vi "VisorTDMS.vi"() -> ()   [LabVIEW 2018]
uses:
  <vilib>/express/express shared/transition.llb/Dynamic To Waveform Array.vi
  <vilib>/express/express signal manip/GetorSetDDTAttributes/Set DDT Attributes/SetT0.vi
  <vilib>/express/express shared/transition.llb/Waveform Array To Dynamic.vi
  <vilib>/express/express signal manip/GetorSetDDTAttributes/Set DDT Attributes/Set DDT Properties.xnode
panel:
  out "fin_video":timestamp
  out "incio_video":timestamp
  out "is_altitude":string
  out "is_heading":string
  out "is_roll":string
  out "is_pitch":string
  out "is_depth":string
  out "is_gps_lon":string
  out "is_gps_lat":string
  out "Frame actual":i64
  in  "Frame-":bool
  in  "Frame+":bool
  in  "Retroceder":bool
  in  "Avanzar":bool
  in  "Mover Frame":i64
  in  "Tab Control":enum32{"TopData", "SubData"}(tab)
  in  "Tab Control 2":T1(tab)
  out "rov_states 2":dbl[](array[numeric])
  out "ind.":dbl[](array[numeric])
  out "modo_ctrl 2":dbl[](array[numeric])
  out "ac_time_TopData":timestamp[](array[timestamp])
  out "gps_alt":dbl[](array[numeric])
  out "usbl_x":dbl[](array[numeric])
  out "usbl_y":dbl[](array[numeric])
  out "usbl_z":dbl[](array[numeric])
  out "vess_ahrs_pitch":dbl[](array[numeric])
  out "vess_ahrs_roll":dbl[](array[numeric])
  out "vess_ahrs_yaw":dbl[](array[numeric])
  out "acquisition_time 5":timestamp[](array[timestamp])
  out "ci_habilitada":dbl[](array[numeric])
  out "CI_Data_joy_1x":dbl[](array[numeric])
  out "CI_Data_jot_1y":dbl[](array[numeric])
  out "CI_Data_jot_1z":dbl[](array[numeric])
  out "CI_Data_joy_1thumb":dbl[](array[numeric])
  out "CI_Data_joy_1botIzq":dbl[](array[numeric])
  out "CI_Data_joy_1botder":dbl[](array[numeric])
  out "acquisition_time 12":timestamp[](array[timestamp])
  out "CI_Data_joy_1gatillo":dbl[](array[numeric])
  out "CI_Data_modo_1bot":dbl[](array[numeric])
  out "CI_Data_modo_2bot":dbl[](array[numeric])
  out "CI_Data_modo_3bot":dbl[](array[numeric])
  out "CI_Data_modo_4bot":dbl[](array[numeric])
  out "CI_Data_pot":dbl[](array[numeric])
  out "CI_Data_enc":dbl[](array[numeric])
  out "CI_Data_joy_2x":dbl[](array[numeric])
  out "CI_Data_joy_2y":dbl[](array[numeric])
  out "CI_Data_joy_2z":dbl[](array[numeric])
  out "CI_Data_joy_2bot":dbl[](array[numeric])
  out "CI_Data_botella_1bot":dbl[](array[numeric])
  out "CI_Data_botella_2bot":dbl[](array[numeric])
  out "CI_Data_botella_3bot":dbl[](array[numeric])
  out "CI_Data_botella_4bot":dbl[](array[numeric])
  out "CI_Data_corer_1bot":dbl[](array[numeric])
  out "CI_Data_corer_2bot":dbl[](array[numeric])
  out "CI_Data_a_in":dbl[](array[numeric])
  out "CI_Data_dio1":dbl[](array[numeric])
  out "CI_Data_dio2":dbl[](array[numeric])
  out "CI_Data_dio3":dbl[](array[numeric])
  out "CI_Data_ci_acc_x":dbl[](array[numeric])
  out "CI_Data_ci_acc_y":dbl[](array[numeric])
  out "CI_Data_ci_acc_z":dbl[](array[numeric])
  out "Surface_Data_modo_1ind":dbl[](array[numeric])
  out "Surface_Data_modo_2ind":dbl[](array[numeric])
  out "Surface_Data_modo_3ind":dbl[](array[numeric])
  out "Surface_Data_modo_4ind":dbl[](array[numeric])
  out "Surface_Data_botella_1ind":dbl[](array[numeric])
  out "Surface_Data_botella_2ind":dbl[](array[numeric])
  out "Surface_Data_botella_3ind":dbl[](array[numeric])
  out "Surface_Data_botella_4ind":dbl[](array[numeric])
  out "Surface_Data_corer_1ind":dbl[](array[numeric])
  out "Surface_Data_corer_2ind":dbl[](array[numeric])
  out "Surface_Data_lars_vel":dbl[](array[numeric])
  out "Surface_Data_lars_fwd":dbl[](array[numeric])
  out "Surface_Data_lars_rev":dbl[](array[numeric])
  out "acquisition_time 13":timestamp[](array[timestamp])
  out "m1_hi":dbl[](array[numeric])
  out "m1_lo":dbl[](array[numeric])
  out "m1_en":dbl[](array[numeric])
  out "m2_hi":dbl[](array[numeric])
  out "m2_lo":dbl[](array[numeric])
  out "m2_en":dbl[](array[numeric])
  out "m3_hi":dbl[](array[numeric])
  out "m3_lo":dbl[](array[numeric])
  out "m3_en":dbl[](array[numeric])
  out "m4_hi":dbl[](array[numeric])
  out "m4_lo":dbl[](array[numeric])
  out "m4_en":dbl[](array[numeric])
  out "m5_hi":dbl[](array[numeric])
  out "m5_lo":dbl[](array[numeric])
  out "m5_en":dbl[](array[numeric])
  out "m6_hi":dbl[](array[numeric])
  out "m6_lo":dbl[](array[numeric])
  out "m6_en":dbl[](array[numeric])
  out "motor_PID_Kp":dbl[](array[numeric])
  out "motor_PID_Ti":dbl[](array[numeric])
  out "motor_PID_Td":dbl[](array[numeric])
  out "m_PID_en":dbl[](array[numeric])
  out "depth_PID_Kp":dbl[](array[numeric])
  out "depth_PID_Ti":dbl[](array[numeric])
  out "depth_PID_Td":dbl[](array[numeric])
  out "depth_sp":dbl[](array[numeric])
  out "heading_PID_Kp":dbl[](array[numeric])
  out "heading_PID_Ti":dbl[](array[numeric])
  out "heading_PID_Td":dbl[](array[numeric])
  out "heading_sp":dbl[](array[numeric])
  out "altitude_PID_Kp":dbl[](array[numeric])
  out "altitude_PID_Ti":dbl[](array[numeric])
  out "altitude_PID_Td":dbl[](array[numeric])
  out "altitude_sp":dbl[](array[numeric])
  out "PID_reset":dbl[](array[numeric])
  out "modo_ctrl":dbl[](array[numeric])
  out "bus_260v":dbl[](array[numeric])
  out "m_1":dbl[](array[numeric])
  out "m_2":dbl[](array[numeric])
  out "m_3":dbl[](array[numeric])
  out "m_4":dbl[](array[numeric])
  out "m_5":dbl[](array[numeric])
  out "m_6":dbl[](array[numeric])
  out "luz_1":dbl[](array[numeric])
  out "luz_2":dbl[](array[numeric])
  out "luz_3":dbl[](array[numeric])
  out "pot_gen":dbl[](array[numeric])
  out "pot_m1":dbl[](array[numeric])
  out "pot_m2":dbl[](array[numeric])
  out "pot_m3":dbl[](array[numeric])
  out "pot_m4":dbl[](array[numeric])
  out "pot_m5":dbl[](array[numeric])
  out "pot_m6":dbl[](array[numeric])
  out "pot_l1":dbl[](array[numeric])
  out "pot_l2":dbl[](array[numeric])
  out "pot_l3":dbl[](array[numeric])
  out "virtual_ci":dbl[](array[numeric])
  out "fuente_muestras":dbl[](array[numeric])
  out "corer_1":dbl[](array[numeric])
  out "corer_2":dbl[](array[numeric])
  out "bot_1":dbl[](array[numeric])
  out "bot_2":dbl[](array[numeric])
  out "bot_3":dbl[](array[numeric])
  out "bot_4":dbl[](array[numeric])
  out "pot_c1":dbl[](array[numeric])
  out "pot_c2":dbl[](array[numeric])
  out "acquisition_time 14":timestamp[](array[timestamp])
  in  "Tab Control 3":T2(tab)
  out "ac_time_SubData":timestamp[](array[timestamp])
  out "sub_ind":dbl[](array[numeric])
  out "sc_ind":dbl[](array[numeric])
  out "rov_states":dbl[](array[numeric])
  out "accel_x":dbl[](array[numeric])
  out "accel_y":dbl[](array[numeric])
  out "accel_z":dbl[](array[numeric])
  out "gyr_x":dbl[](array[numeric])
  out "acquisition_time 2":timestamp[](array[timestamp])
  out "gyr_y":dbl[](array[numeric])
  out "gyr_z":dbl[](array[numeric])
  out "mag_x":dbl[](array[numeric])
  out "mag_y":dbl[](array[numeric])
  out "mag_z":dbl[](array[numeric])
  out "acquisition_time 4":timestamp[](array[timestamp])
  out "pressure 4":dbl[](array[numeric])
  out "temperature 4":dbl[](array[numeric])
  out "conductivity":dbl[](array[numeric])
  out "density":dbl[](array[numeric])
  out "salinity":dbl[](array[numeric])
  out "speed_of_sound":dbl[](array[numeric])
  out "acquisition_time 3":timestamp[](array[timestamp])
  out "acquisition_time 6":timestamp[](array[timestamp])
  out "liquid_smp1":dbl[](array[numeric])
  out "liquid_smp2":dbl[](array[numeric])
  out "liquid_smp3":dbl[](array[numeric])
  out "liquid_smp4":dbl[](array[numeric])
  out "solid_smp1":dbl[](array[numeric])
  out "solid_smp2":dbl[](array[numeric])
  out "supply_12V":dbl[](array[numeric])
  out "motor_signal1":dbl[](array[numeric])
  out "motor_signal2":dbl[](array[numeric])
  out "cur_liq_1":dbl[](array[numeric])
  out "cur_liq_2":dbl[](array[numeric])
  out "ac_status":dbl[](array[numeric])
  out "voltaje_hvdc":dbl[](array[numeric])
  out "current_hvdc":dbl[](array[numeric])
  out "light1":dbl[](array[numeric])
  out "light2":dbl[](array[numeric])
  out "ligth_sphere":dbl[](array[numeric])
  out "voltage_l1_l2":dbl[](array[numeric])
  out "voltage_l2_l3":dbl[](array[numeric])
  out "voltage_l1_l3":dbl[](array[numeric])
  out "current_l1":dbl[](array[numeric])
  out "current_l2":dbl[](array[numeric])
  out "current_l3":dbl[](array[numeric])
  out "acquisition_time 7":timestamp[](array[timestamp])
  out "current_lights":dbl[](array[numeric])
  out "temp_ac_filter":dbl[](array[numeric])
  out "MA_1_status":dbl[](array[numeric])
  out "MA_1_ctr_signal":dbl[](array[numeric])
  out "MA_1_current":dbl[](array[numeric])
  out "MA_1_speed":dbl[](array[numeric])
  out "MA_2_status":dbl[](array[numeric])
  out "MA_2_ctr_signal":dbl[](array[numeric])
  out "MA_2_current":dbl[](array[numeric])
  out "MA_2_speed":dbl[](array[numeric])
  out "MA_3_status":dbl[](array[numeric])
  out "MA_3_ctr_signal":dbl[](array[numeric])
  out "MA_3_current":dbl[](array[numeric])
  out "MA_3_speed":dbl[](array[numeric])
  out "MA_4_status":dbl[](array[numeric])
  out "MA_4_ctr_signal":dbl[](array[numeric])
  out "MA_4_current":dbl[](array[numeric])
  out "MA_4_speed":dbl[](array[numeric])
  out "MA_5_status":dbl[](array[numeric])
  out "MA_5_ctr_signal":dbl[](array[numeric])
  out "MA_5_current":dbl[](array[numeric])
  out "MA_5_speed":dbl[](array[numeric])
  out "MA_6_status":dbl[](array[numeric])
  out "MA_6_ctr_signal":dbl[](array[numeric])
  out "MA_6_current":dbl[](array[numeric])
  out "MA_6_speed":dbl[](array[numeric])
  out "mode":dbl[](array[numeric])
  out "start":dbl[](array[numeric])
  out "lps":dbl[](array[numeric])
  out "controller":dbl[](array[numeric])
  out "voltage":dbl[](array[numeric])
  out "current":dbl[](array[numeric])
  out "temperature":dbl[](array[numeric])
  out "humidity":dbl[](array[numeric])
  out "leak":dbl[](array[numeric])
  out "pressure":dbl[](array[numeric])
  out "acquisition_time 8":timestamp[](array[timestamp])
  out "mode 2":dbl[](array[numeric])
  out "start 2":dbl[](array[numeric])
  out "lps 2":dbl[](array[numeric])
  out "controller 2":dbl[](array[numeric])
  out "voltage 2":dbl[](array[numeric])
  out "current 2":dbl[](array[numeric])
  out "temperature 2":dbl[](array[numeric])
  out "humidity 2":dbl[](array[numeric])
  out "leak 2":dbl[](array[numeric])
  out "pressure 2":dbl[](array[numeric])
  out "acquisition_time 9":timestamp[](array[timestamp])
  out "mode 3":dbl[](array[numeric])
  out "start 3":dbl[](array[numeric])
  out "lps 3":dbl[](array[numeric])
  out "controller 3":dbl[](array[numeric])
  out "voltage 3":dbl[](array[numeric])
  out "current 3":dbl[](array[numeric])
  out "temperature 3":dbl[](array[numeric])
  out "humidity 3":dbl[](array[numeric])
  out "leak 3":dbl[](array[numeric])
  out "pressure 3":dbl[](array[numeric])
  out "acquisition_time 10":timestamp[](array[timestamp])
  out "ctrl_state":dbl[](array[numeric])
  out "rov_output_x":dbl[](array[numeric])
  out "rov_output_y":dbl[](array[numeric])
  out "rov_output_z":dbl[](array[numeric])
  out "rov_output_yaw":dbl[](array[numeric])
  out "dac_outputs":dbl[](array[numeric])
  out "in_range":dbl[](array[numeric])
  out "motor_ctrl_array_setpoint":dbl[](array[numeric])
  out "motor_ctrl_array_sensor":dbl[](array[numeric])
  out "acquisition_time 11":timestamp[](array[timestamp])
  in  "saving":bool
  in  "view SubData":bool
  in  "view TopData":bool
  in  "save data":bool
  in  "Path TopData":path
  out "gps_lon":dbl[](array[numeric])
  out "gps_lat":dbl[](array[numeric])
  out "inicio_TopData":timestamp
  out "fin_TopData":timestamp
  out "round_ac_time_TopData":timestamp[](array[timestamp])
  out "round_ac_time_SubData":timestamp[](array[timestamp])
  out "round Time Stamp":timestamp
  in  "Path .avi":path
  out "fin_SubData":timestamp
  out "inicio_SubData":timestamp
  in  "Path SubData":path
  out "depth":dbl[](array[numeric])
  in  "timestamp LabVIEW":dbl format="%#.7f"
  out "Time stamp video":timestamp
  out "altitude":dbl[](array[numeric])
  out "heading":dbl[](array[numeric])
  out "roll":dbl[](array[numeric])
  out "pitch":dbl[](array[numeric])
  in  "Slide":i64(slide) min=0 max=52348 scale=0.0..52348.0
  out "Video":T3(plugin-control)
  in  "stop":bool
  # "Requisitos VI:\n*Video en formato AVI\n*No correr el VI desde una carpeta sincronizada en nube (OneDrive), puede generar errores al momento de sobre escribir el .xlsx generado dado que el archivo es usado en segundo plano para la sincronización de la nube en cuestión"
  # "Status"
  # "DAQ"
  # "User_Data"
  # "Virtual_CI"
  # "Control"
  # "Status"
  # "AHRS"
  # "CTD"
  # "ALTIMETER"
  # "SMP"
  # "PWR"
  # "SC_PWR"
  # "SC_CPU"
  # "SC_SMP"
  # "Control"
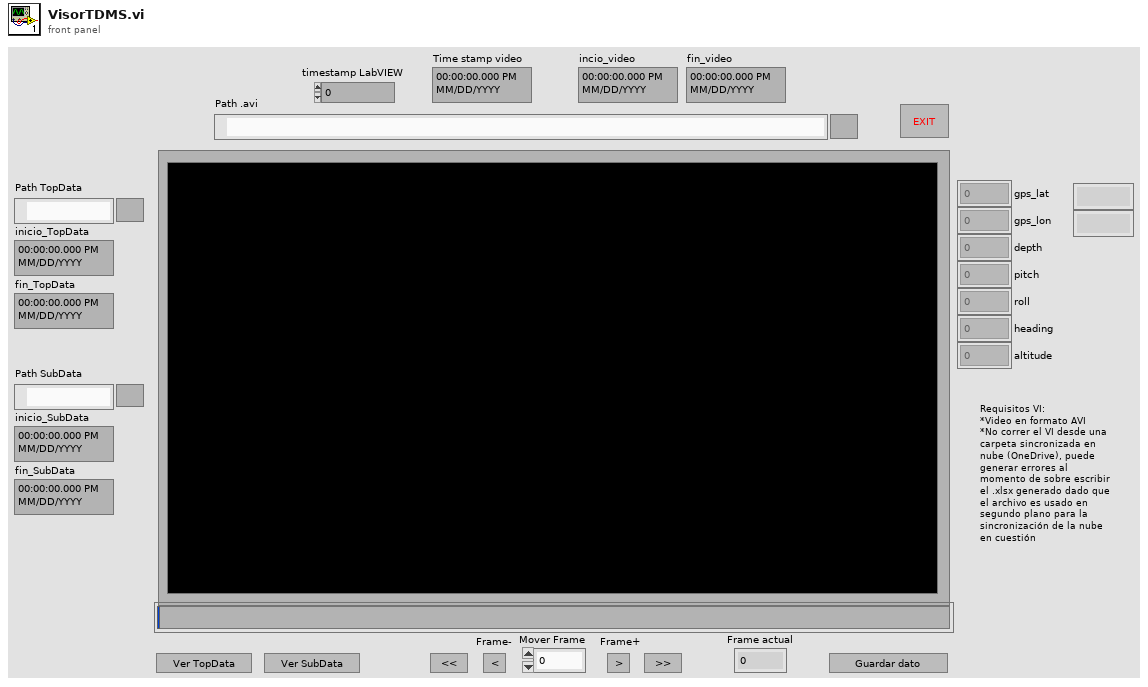
[diagram p1: front panel]
types:
  T1 = enum32{"Status", "DAQ", "User_Data", "Virtual_CI", "Control"}
  T2 = enum32{"Status", "AHRS", "CTD", "ALTIMETER", "SMP", "PWR", "SC_PWR", "SC_CPU", "SC_SMP", "Control"}
  T3 = typedef "IMAQ Image.ctl" = refnum<image>
  T4 = typedef "AviRefnum.ctl" = refnum<k1>
  T5 = typedef "Image Type" = u32
  T6 = enum8{"Enabled", "Disabled", "Disabled and Grayed Out"}
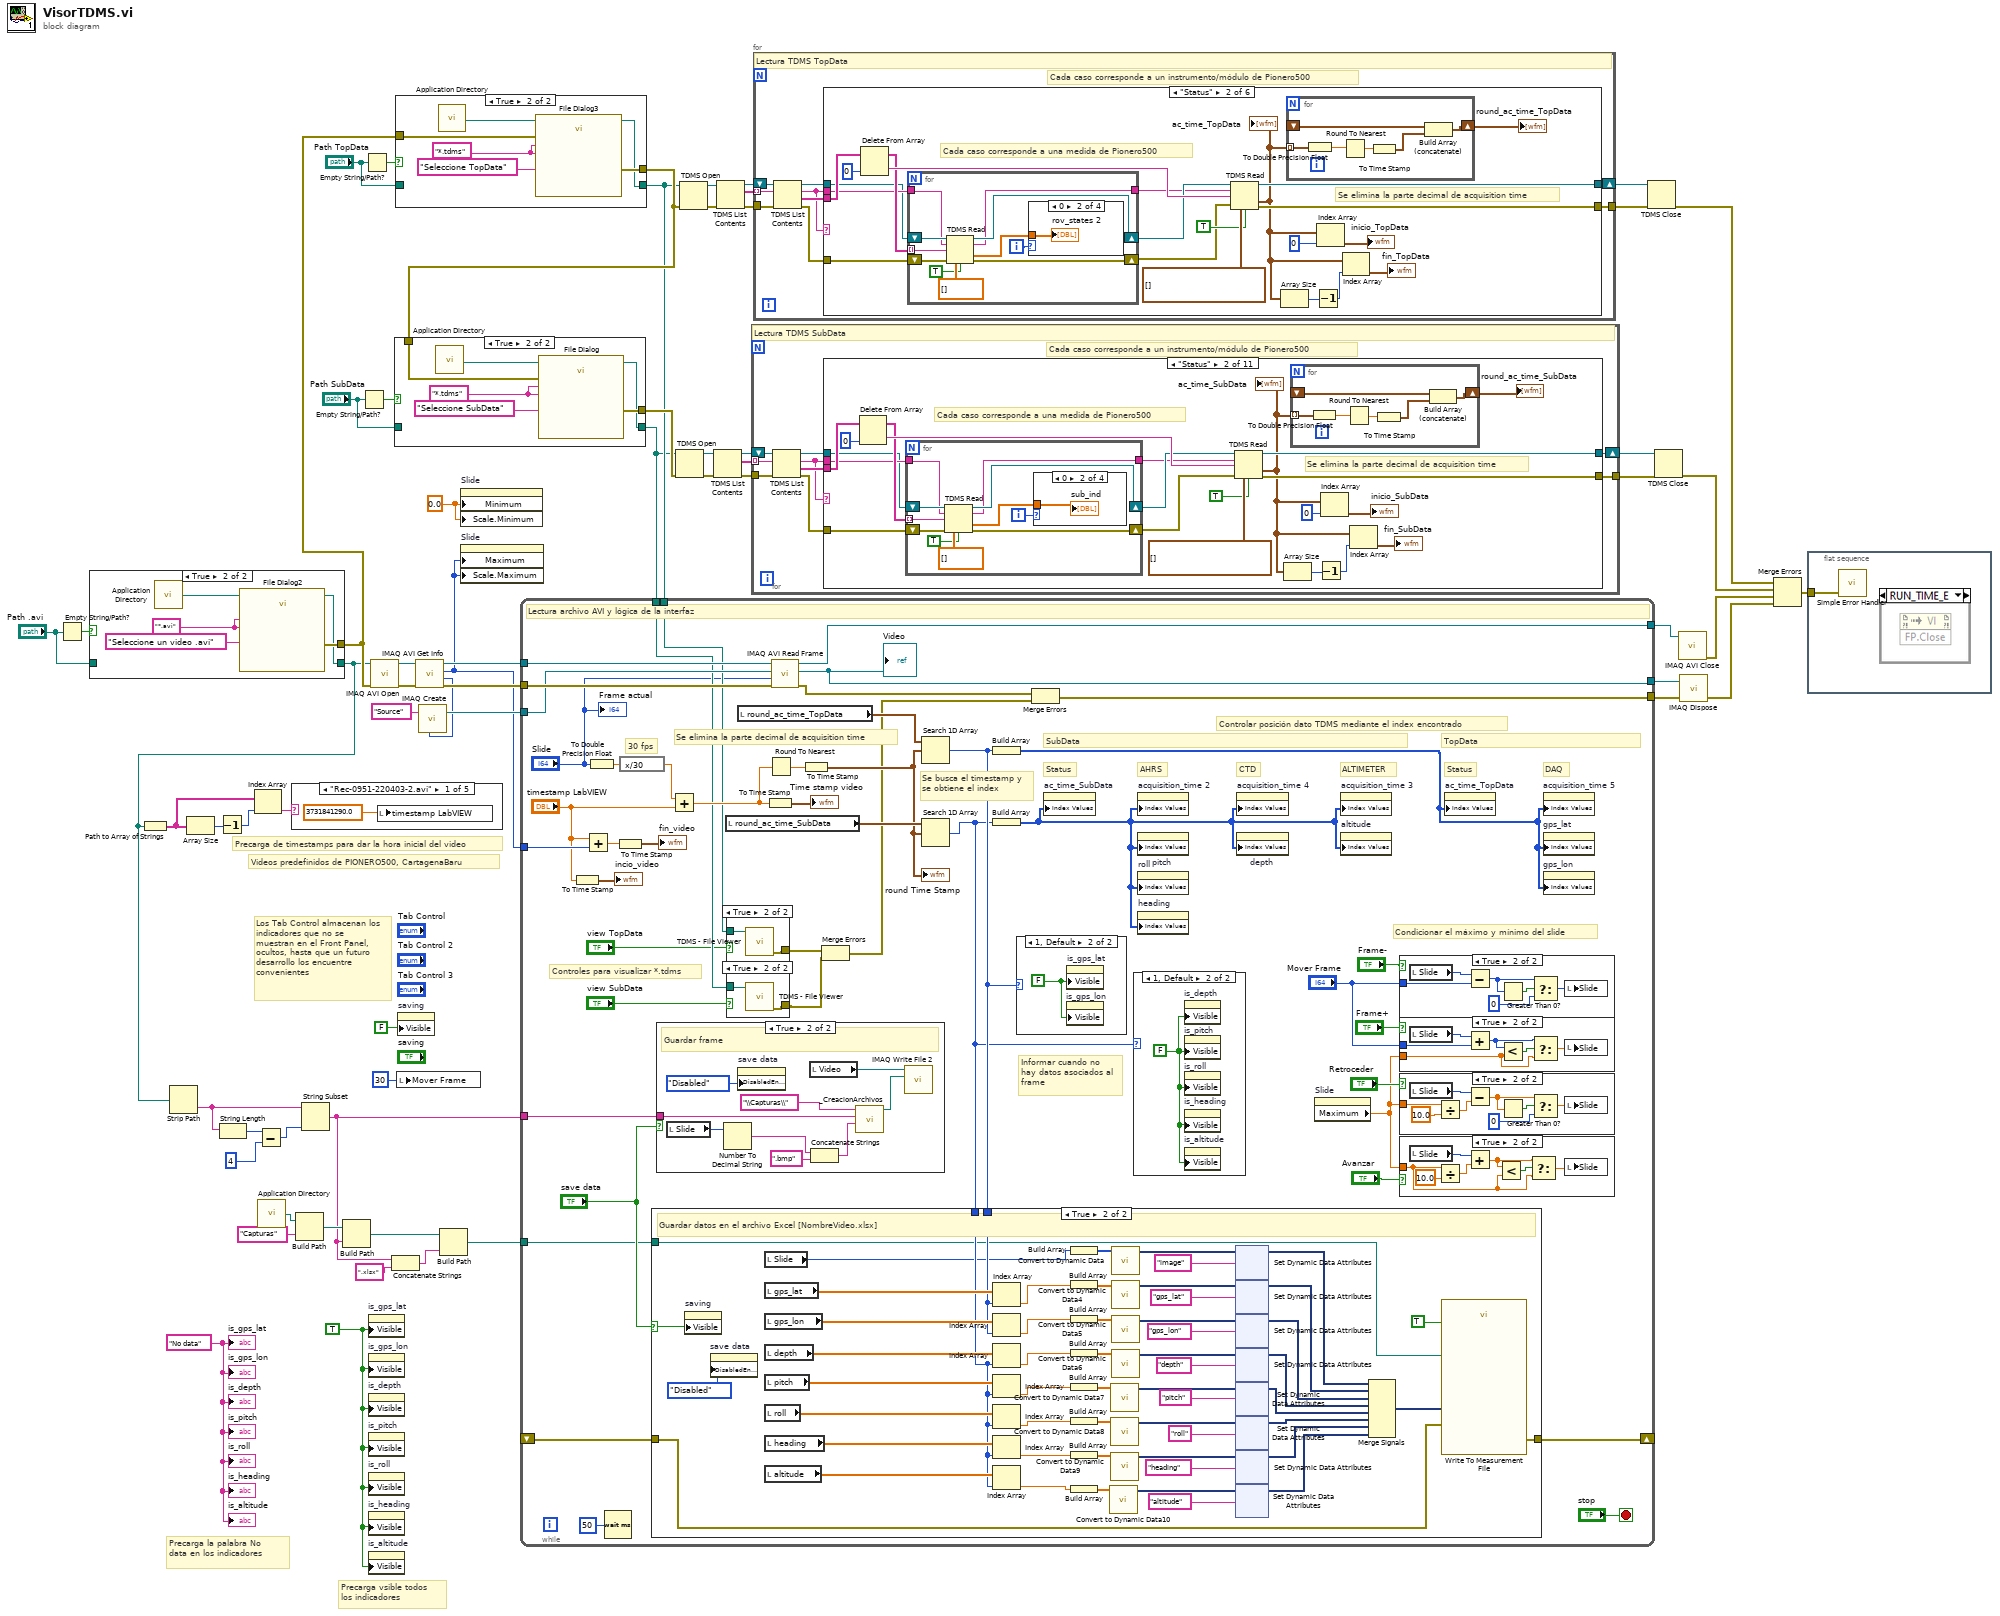
[diagram p0: block diagram]
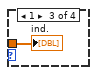
[diagram p5: hidden frame]
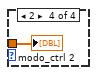
[diagram p6: hidden frame]
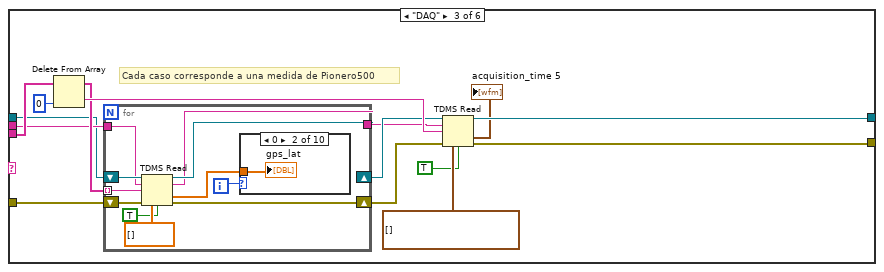
[diagram p7: hidden frame]
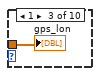
[diagram p9: hidden frame]
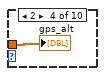
[diagram p10: hidden frame]
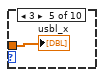
[diagram p11: hidden frame]
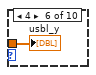
[diagram p12: hidden frame]
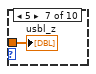
[diagram p13: hidden frame]
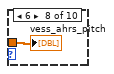
[diagram p14: hidden frame]
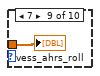
[diagram p15: hidden frame]
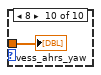
[diagram p16: hidden frame]
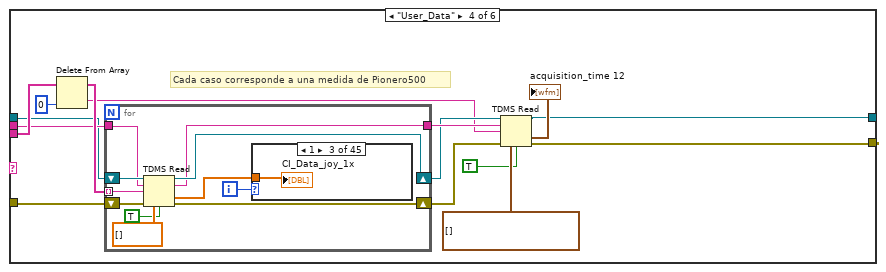
[diagram p17: hidden frame]
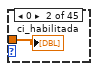
[diagram p19: hidden frame]
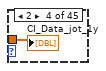
[diagram p20: hidden frame]
diagram:
  w3 = TRUE ("Visible")
  w2 = "No data" ("is_gps_lat")
  w6 = 0.0 ("Data Entry Limits:Minimum")
  # "Los Tab Control almacenan los indicadores que no se muestran en el Front Panel, ocultos, hasta que un futuro desarrollo los encuentre convenientes"
  # "Precarga vsible todos los indicadores"
  # "Precarga la palabra No data en los indicadores"
  # "Videos predefinidos de PIONERO500, CartagenaBaru"
  # "Precarga de timestamps para dar la hora inicial del video"
  n1 = Empty String/Path?(string/path="Path .avi") -> (empty?=w48:bool)
  n2 = case shown="True" w48 {
    tunnel: [_ w69] -> w26
    tunnel: [w64 w68] -> w17
    tunnel: "Path .avi" -> [w64 _]
    frame False {
    }
    frame True {
      w66 = "*.avi" ("pattern (all files)")
      n3 = call <vilib>:"Application Directory.vi"() -> ("Application Directory"=w65:path)
      n4 = call "File Dialog2"("start path"=w65, "prompt"="Seleccione un video .avi", "pattern (all files)"=w66, "pattern label"=w66) -> ("selected path"=w68:path, "error out"=w69:errorcluster)  [unwired: 8 in, 2 out]
    }
  }
  n5 = Path to Array of Strings(0:w17) -> (2:w53:string[])  [unwired: 1 out]
  n6 = Strip Path(path=w17) -> (name=w16:string)  [unwired: 1 out]
  n7 = Array Size(array=w53) -> (size(s)=w54:i32)
  n8 = Decrement(x=w54) -> (x-1=w25:i32)
  n9 = String Length(string=w16) -> (length=w20:i32)
  n10 = Index Array(array=w53, index=w25) -> (element=w52:string)
  n11 = Subtract(x=w20, y=4) -> (x-y=w18:i32)
  n12 = call <vilib>:"Application Directory.vi"() -> ("Application Directory"=w14:path)
  n13 = case shown="\"Rec-0951-220403-2.avi\"" w52 {
    frame "Rec-0951-220403-2.avi" {
      n14 = local write "timestamp LabVIEW"(3731841290.0 ("timestamp DIAdem")) -> ()
    }
    frame "Rec-1224-220403-9.avi" {
      n15 = local write "timestamp LabVIEW"(3731850459.0 ("timestamp DIAdem")) -> ()
    }
    frame "Rec-1421-220403-12.avi" {
      n16 = local write "timestamp LabVIEW"(3731857520.0 ("timestamp DIAdem")) -> ()
    }
    frame "Rec-1539-220403-19.avi" {
      n17 = local write "timestamp LabVIEW"(3731862092.0 ("timestamp DIAdem")) -> ()
    }
    frame Default {
      n18 = local write "timestamp LabVIEW"(0.0 ("timestamp DIAdem")) -> ()
    }
  }
  n19 = Build Path(base path=w14, name or relative path="Capturas") -> (appended path=w12:path)
  n20 = String Subset(string=w16, length (rest)=w18) -> (substring=w9:string)  [unwired: 1 in]
  n21 = Build Path(base path=w12, name or relative path=w9) -> (appended path=w11:path)
  n22 = Empty String/Path?(string/path="Path SubData") -> (empty?=w39:bool)
  n23 = Empty String/Path?(string/path="Path TopData") -> (empty?=w29:bool)
  n24 = property on="is_gps_lat" class="Str"("Visible"=w3) -> ()  [unwired: 2 in, 2 out]
  n25 = property on="is_gps_lon" class="Str"("Visible"=w3) -> ()  [unwired: 2 in, 2 out]
  n26 = property on="is_depth" class="Str"("Visible"=w3) -> ()  [unwired: 2 in, 2 out]
  n27 = property on="is_pitch" class="Str"("Visible"=w3) -> ()  [unwired: 2 in, 2 out]
  n28 = property on="is_roll" class="Str"("Visible"=w3) -> ()  [unwired: 2 in, 2 out]
  n29 = property on="is_heading" class="Str"("Visible"=w3) -> ()  [unwired: 2 in, 2 out]
  n30 = property on="is_altitude" class="Str"("Visible"=w3) -> ()  [unwired: 2 in, 2 out]
  n31 = call "IMAQ AVI Open"("error in (no error)"=w26, "AVI Path"=w17) -> ("error out"=w59:errorcluster, "Avi Refnum"=w56:T4)  [unwired: 8 in]
  n32 = Concatenate Strings(w9, ".xlsx" ("string")) -> (w8:string)
  n33 = case shown="True" w29 {
    tunnel: [_ w81] -> w28
    tunnel: [w75 w80] -> w22
    tunnel: "Path TopData" -> [w75 _]
    tunnel: w26 -> [_ w76]
    frame False {
    }
    frame True {
      w77 = "*.tdms" ("pattern (all files)")
      n34 = call <vilib>:"Application Directory.vi"() -> ("Application Directory"=w78:path)
      n35 = call "File Dialog3"("start path"=w78, "prompt"="Seleccione TopData", "error in"=w76, "pattern (all files)"=w77, "pattern label"=w77) -> ("selected path"=w80:path, "error out"=w81:errorcluster)  [unwired: 7 in, 2 out]
    }
  }
  n36 = case shown="True" w39 {
    tunnel: [_ w88] -> w27
    tunnel: [w82 w87] -> w21
    tunnel: "Path SubData" -> [w82 _]
    tunnel: w28 -> [_ w83]
    frame False {
    }
    frame True {
      w84 = "*.tdms" ("pattern (all files)")
      n37 = call <vilib>:"Application Directory.vi"() -> ("Application Directory"=w85:path)
      n38 = call "File Dialog"("start path"=w85, "prompt"="Seleccione SubData", "error in"=w83, "pattern (all files)"=w84, "pattern label"=w84) -> ("selected path"=w87:path, "error out"=w88:errorcluster)  [unwired: 7 in, 2 out]
    }
  }
  n39 = local write "Mover Frame"(i64 30 ("Mover Frame")) -> ()
  n40 = property on="saving" class="Bool"("Visible"=FALSE) -> ()  [unwired: 2 in, 2 out]
  n41 = call "IMAQ AVI Get Info"("error in (no error)"=w59, "Avi Refnum"=w56) -> ("error out"=w58:errorcluster, "Image Type"=w55:T5, "Number of Frames"=w1:u32, "Avi Refnum (duplicate)"=w57:T4)  [unwired: 5 in, 1 out]
  n42 = call "IMAQ Create"("Image Name"="Source", "Image Type"=w55) -> ("New Image"=w62:T3)  [unwired: 3 in, 1 out]
  n43 = Build Path(base path=w11, name or relative path=w8) -> (appended path=w7:path)
  n44 = property on="Slide" class="Slide (strict)"("Minimum"=w6, "Scale.Minimum"=w6) -> ()  [unwired: 2 in, 2 out]
  n45 = property on="Slide" class="Slide (strict)"("Maximum"=w1, "Scale.Maximum"=w1) -> ()  [unwired: 2 in, 2 out]
  n46 = while {
    tunnel: w58 -> [w133]
    tunnel: [w132] -> w63
    tunnel: w57 -> [w131]
    tunnel: w62 -> [w130]
    tunnel: [w101] -> w60
    tunnel: w22 -> [w118]
    tunnel: w21 -> [w117]
    tunnel: w9 -> [w112]
    shift-right: [w111] -> _
    shift-left: _ -> [w110]
    tunnel: w7 -> [w109]
    tunnel: [w96] -> w4
    tunnel: w1 -> [w90]
    stop <- "stop" stop-if-true
    # "Se elimina la parte decimal de acquisition time"
    # "Se busca el timestamp y se obtiene el index"
    # "Informar cuando no hay datos asociados al frame"
    # "Condicionar el máximo y mínimo del slide"
    # "Controles para visualizar *.tdms"
    # "TopData"
    # "DAQ"
    # "Status"
    # "SubData"
    # "ALTIMETER"
    # "CTD"
    # "AHRS"
    # "Status"
    # "30 fps"
    # "Controlar posición dato TDMS mediante el index encontrado"
    # "Lectura archivo AVI y lógica de la interfaz"
    n47 = To Time Stamp(1:"timestamp LabVIEW") -> (0:→"incio_video":timestamp)
    n48 = Add(x="timestamp LabVIEW", y=w90) -> (x+y=w91:dbl)
    n49 = To Double Precision Float(number="Slide") -> (double precision float=w127:dbl)
    n50 = Wait (ms)(milliseconds to wait=u32 50) -> ()  [unwired: 1 out]
    n51 = To Time Stamp(1:w91) -> (0:→"fin_video":timestamp)
    n52 = expression code="x/30"(w127) -> (w128:dbl)
    n53 = case shown="True" "save data" {
      tunnel: w112 -> [_ w170]
      frame False {
        # "Guardando frame (espera guardar frame)"
        n54 = property on="save data" class="Bool"("DisabledEnum"=T6."Enabled" ("Disabled")) -> ()  [unwired: 2 in, 2 out]
      }
      frame True {
        # "Guardar frame"
        n55 = local read "Slide"() -> (w168:i64)
        n56 = Number To Decimal String(number=w168) -> (decimal integer string=w167:string)  [unwired: 1 in]
        n57 = property on="save data" class="Bool"("DisabledEnum"=T6."Disabled" ("Disabled")) -> ()  [unwired: 2 in, 2 out]
        n58 = local read "Video"() -> (w174:T3)
        n59 = Concatenate Strings(w167, ".bmp" ("string")) -> (w169:string)
        n60 = call "_CreacionArchivos.vi"("Tipo_Data"=w169, "Nombre_mision"=w170, "Carpeta"="\\Capturas\\" ("element")) -> ("appended path"=w172:path)  [unwired: 8 in]
        n61 = call-poly "IMAQ Write File 2"("File Path"=w172, "Image"=w174) -> ()  [unwired: 8 in, 2 out]
      }
    }
    n62 = Add(x=w128, y="timestamp LabVIEW") -> (x+y=w124:dbl)
    n63 = local read "round_ac_time_SubData"() -> (w122:timestamp[])
    n64 = case shown="True" "view TopData" {
      tunnel: w118 -> [_ w349]
      tunnel: [_ w348] -> w98
      frame False {
      }
      frame True {
        n65 = call <vilib>:"TDMS - File Viewer.vi"("file path"=w349) -> ("error out"=w348:errorcluster)  [unwired: 5 in, 1 out]
      }
    }
    n66 = case shown="True" "view SubData" {
      tunnel: w117 -> [_ w347]
      tunnel: [_ w346] -> w99
      frame False {
      }
      frame True {
        n67 = call <vilib>:"TDMS - File Viewer.vi"("file path"=w347) -> ("error out"=w346:errorcluster)  [unwired: 5 in, 1 out]
      }
    }
    n68 = local read "round_ac_time_TopData"() -> (w121:timestamp[])
    n69 = To Time Stamp(1:w124) -> (0:→"Time stamp video":timestamp)
    n70 = Round To Nearest(number=w124) -> (nearest integer value=w125:dbl)
    n71 = call "IMAQ AVI Read Frame"("error in (no error)"=w133, "Frame Number"="Slide", "Image"=w130, "Avi Refnum"=w131) -> ("error out"=w100:errorcluster, "Image Out"=w101:T3, "Avi Refnum (duplicate)"=w132:T4)  [unwired: 4 in, 1 out]
    "Video" <- w101
    n72 = To Time Stamp(1:w125) -> (0:w120:timestamp)
    "round Time Stamp" <- w120
    n73 = Merge Errors(w98, w99) -> (w97:errorcluster)
    n74 = Search 1D Array(1D array=w121, element=w120) -> (index of element=w95:i32)  [unwired: 1 in]
    n75 = Search 1D Array(1D array=w122, element=w120) -> (index of element=w94:i32)  [unwired: 1 in]
    n76 = case shown="True" "save data" {
      selector: "save data" -> [w176 w180]
      tunnel: w95 -> [_ w226]
      tunnel: w94 -> [_ w225]
      tunnel: [w177 w182] -> w111
      tunnel: w110 -> [w177 w181]
      tunnel: w109 -> [_ w179]
      frame False {
        # "Guardando dato (espera guardar dato en *.xlsx)"
        n77 = property on="saving" class="Bool"("Visible"=w176) -> ()  [unwired: 2 in, 2 out]
        n78 = property on="save data" class="Bool"("DisabledEnum"=T6."Enabled" ("Disabled")) -> ()  [unwired: 2 in, 2 out]
      }
      frame True {
        # "Guardar datos en el archivo Excel [NombreVideo.xlsx]"
        n79 = property on="saving" class="Bool"("Visible"=w180) -> ()  [unwired: 2 in, 2 out]
        n80 = property on="save data" class="Bool"("DisabledEnum"=T6."Disabled" ("Disabled")) -> ()  [unwired: 2 in, 2 out]
        n81 = local read "Slide"() -> (w190:i64)
        n82 = local read "gps_lat"() -> (w233:dbl[])
        n83 = local read "gps_lon"() -> (w232:dbl[])
        n84 = local read "depth"() -> (w231:dbl[])
        n85 = local read "pitch"() -> (w230:dbl[])
        n86 = local read "roll"() -> (w229:dbl[])
        n87 = local read "heading"() -> (w228:dbl[])
        n88 = local read "altitude"() -> (w227:dbl[])
        n89 = Index Array(array=w233, index=w226) -> (element=w191:dbl)
        n90 = Index Array(array=w232, index=w226) -> (element=w192:dbl)
        n91 = Index Array(array=w231, index=w225) -> (element=w193:dbl)
        n92 = Index Array(array=w230, index=w225) -> (element=w194:dbl)
        n93 = Index Array(array=w229, index=w225) -> (element=w195:dbl)
        n94 = Index Array(array=w228, index=w225) -> (element=w196:dbl)
        n95 = Index Array(array=w227, index=w225) -> (element=w197:dbl)
        n96 = Build Array(w190) -> (w189:i64[])
        n97 = Build Array(w191) -> (w188:dbl[])
        n98 = Build Array(w192) -> (w187:dbl[])
        n99 = Build Array(w193) -> (w186:dbl[])
        n100 = Build Array(w194) -> (w185:dbl[])
        n101 = Build Array(w195) -> (w184:dbl[])
        n102 = Build Array(w196) -> (w183:dbl[])
        n103 = Build Array(w197) -> (w198:dbl[])
        n104 = call "Convert to Dynamic Data10"("Array"=w198) -> ("Dynamic Data Type"=w218:dynamicdata)  [unwired: 3 in]
        n105 = call "Convert to Dynamic Data7"("Array"=w185) -> ("Dynamic Data Type"=w215:dynamicdata)  [unwired: 3 in]
        n106 = call "Convert to Dynamic Data8"("Array"=w184) -> ("Dynamic Data Type"=w216:dynamicdata)  [unwired: 3 in]
        n107 = call "Convert to Dynamic Data9"("Array"=w183) -> ("Dynamic Data Type"=w217:dynamicdata)  [unwired: 3 in]
        n108 = call "Convert to Dynamic Data"("Array"=w189) -> ("Dynamic Data Type"=w223:dynamicdata)  [unwired: 3 in]
        n109 = call "Convert to Dynamic Data4"("Array"=w188) -> ("Dynamic Data Type"=w209:dynamicdata)  [unwired: 3 in]
        n110 = call "Convert to Dynamic Data5"("Array"=w187) -> ("Dynamic Data Type"=w210:dynamicdata)  [unwired: 3 in]
        n111 = call "Convert to Dynamic Data6"("Array"=w186) -> ("Dynamic Data Type"=w213:dynamicdata)  [unwired: 3 in]
        n112 = xnode ("Set Dynamic Data Attributes")("Signals In"=w223, "Signal Name"="image") -> ("Signals Out"=w224:dynamicdata)  [unwired: 2 in, 1 out]
        n113 = xnode ("Set Dynamic Data Attributes")("Signals In"=w209, "Signal Name"="gps_lat") -> ("Signals Out"=w212:dynamicdata)  [unwired: 2 in, 1 out]
        n114 = xnode ("Set Dynamic Data Attributes")("Signals In"=w210, "Signal Name"="gps_lon") -> ("Signals Out"=w211:dynamicdata)  [unwired: 2 in, 1 out]
        n115 = xnode ("Set Dynamic Data Attributes")("Signals In"=w213, "Signal Name"="depth") -> ("Signals Out"=w214:dynamicdata)  [unwired: 2 in, 1 out]
        n116 = xnode ("Set Dynamic Data Attributes")("Signals In"=w215, "Signal Name"="pitch") -> ("Signals Out"=w219:dynamicdata)  [unwired: 2 in, 1 out]
        n117 = xnode ("Set Dynamic Data Attributes")("Signals In"=w216, "Signal Name"="roll") -> ("Signals Out"=w220:dynamicdata)  [unwired: 2 in, 1 out]
        n118 = xnode ("Set Dynamic Data Attributes")("Signals In"=w217, "Signal Name"="heading") -> ("Signals Out"=w221:dynamicdata)  [unwired: 2 in, 1 out]
        n119 = xnode ("Set Dynamic Data Attributes")("Signals In"=w218, "Signal Name"="altitude") -> ("Signals Out"=w222:dynamicdata)  [unwired: 2 in, 1 out]
        n120 = Merge Signals(w224, w212, w211, w214, w219, w220, w221, w222) -> (w208:dynamicdata)
        n121 = call "Write To Measurement File"("Signals"=w208, "Enable"=TRUE, "error in (no error)"=w181, "Filename"=w179) -> ("error out"=w182:errorcluster)  [unwired: 13 in, 2 out]
      }
    }
    n122 = Build Array(w95) -> (w119:i32[])
    n123 = Build Array(w94) -> (w126:i32[])
    n124 = case shown="1, Default" w95 {
      frame -1 {
        w136 = TRUE ("Visible")
        n125 = property on="is_gps_lat" class="Str"("Visible"=w136) -> ()  [unwired: 2 in, 2 out]
        n126 = property on="is_gps_lon" class="Str"("Visible"=w136) -> ()  [unwired: 2 in, 2 out]
      }
      frame 1, Default {
        w137 = FALSE ("Visible")
        n127 = property on="is_gps_lat" class="Str"("Visible"=w137) -> ()  [unwired: 2 in, 2 out]
        n128 = property on="is_gps_lon" class="Str"("Visible"=w137) -> ()  [unwired: 2 in, 2 out]
      }
    }
    n129 = Merge Errors(w100, w97) -> (w96:errorcluster)
    n130 = property on="ac_time_SubData" class="Arr (strict)"("Index Values"=w126) -> ()  [unwired: 2 in, 2 out]
    n131 = case shown="1, Default" w94 {
      frame -1 {
        w134 = TRUE ("Visible")
        n132 = property on="is_depth" class="Str"("Visible"=w134) -> ()  [unwired: 2 in, 2 out]
        n133 = property on="is_pitch" class="Str"("Visible"=w134) -> ()  [unwired: 2 in, 2 out]
        n134 = property on="is_roll" class="Str"("Visible"=w134) -> ()  [unwired: 2 in, 2 out]
        n135 = property on="is_heading" class="Str"("Visible"=w134) -> ()  [unwired: 2 in, 2 out]
        n136 = property on="is_altitude" class="Str"("Visible"=w134) -> ()  [unwired: 2 in, 2 out]
      }
      frame 1, Default {
        w135 = FALSE ("Visible")
        n137 = property on="is_depth" class="Str"("Visible"=w135) -> ()  [unwired: 2 in, 2 out]
        n138 = property on="is_pitch" class="Str"("Visible"=w135) -> ()  [unwired: 2 in, 2 out]
        n139 = property on="is_roll" class="Str"("Visible"=w135) -> ()  [unwired: 2 in, 2 out]
        n140 = property on="is_heading" class="Str"("Visible"=w135) -> ()  [unwired: 2 in, 2 out]
        n141 = property on="is_altitude" class="Str"("Visible"=w135) -> ()  [unwired: 2 in, 2 out]
      }
    }
    n142 = property on="acquisition_time 2" class="Arr (strict)"("Index Values"=w126) -> ()  [unwired: 2 in, 2 out]
    n143 = property on="pitch" class="Arr (strict)"("Index Values"=w126) -> ()  [unwired: 2 in, 2 out]
    n144 = property on="roll" class="Arr (strict)"("Index Values"=w126) -> ()  [unwired: 2 in, 2 out]
    n145 = property on="heading" class="Arr (strict)"("Index Values"=w126) -> ()  [unwired: 2 in, 2 out]
    n146 = property on="acquisition_time 4" class="Arr (strict)"("Index Values"=w126) -> ()  [unwired: 2 in, 2 out]
    n147 = property on="depth" class="Arr (strict)"("Index Values"=w126) -> ()  [unwired: 2 in, 2 out]
    n148 = property on="Slide" class="Slide (strict)"() -> ("Maximum"=w102:dbl)  [unwired: 2 in, 2 out]
    n149 = property on="acquisition_time 3" class="Arr (strict)"("Index Values"=w126) -> ()  [unwired: 2 in, 2 out]
    n150 = property on="altitude" class="Arr (strict)"("Index Values"=w126) -> ()  [unwired: 2 in, 2 out]
    n151 = case shown="True" "Frame-" {
      tunnel: "Mover Frame" -> [_ w163]
      frame False {
      }
      frame True {
        n152 = local read "Slide"() -> (w164:i64)
        n153 = Subtract(x=w164, y=w163) -> (x-y=w161:i64)
        n154 = Greater Than 0?(x=w161) -> (x > 0?=w162:bool)
        n155 = Select(t=w161, s=w162, f=i64 0) -> (s? t:f=w160:i64)
        n156 = local write "Slide"(w160) -> ()
      }
    }
    n157 = case shown="True" "Frame+" {
      tunnel: "Mover Frame" -> [_ w157]
      tunnel: w102 -> [_ w153]
      frame False {
      }
      frame True {
        n158 = local read "Slide"() -> (w158:i64)
        n159 = Add(x=w158, y=w157) -> (x+y=w154:i64)
        n160 = Less?(x=w154, y=w153) -> (x < y?=w156:bool)
        n161 = Select(t=w154, s=w156, f=w153) -> (s? t:f=w155:dbl)
        n162 = local write "Slide"(w155) -> ()
      }
    }
    n163 = case shown="True" "Retroceder" {
      tunnel: w102 -> [_ w149]
      frame False {
      }
      frame True {
        n164 = local read "Slide"() -> (w152:i64)
        n165 = Divide(x=w149, y=10.0) -> (x/y=w150:dbl)
        n166 = Subtract(x=w152, y=w150) -> (x-y=w146:dbl)
        n167 = Greater Than 0?(x=w146) -> (x > 0?=w147:bool)
        n168 = Select(t=w146, s=w147, f=i64 0) -> (s? t:f=w145:dbl)
        n169 = local write "Slide"(w145) -> ()
      }
    }
    n170 = case shown="True" "Avanzar" {
      tunnel: w102 -> [_ w139]
      frame False {
      }
      frame True {
        n171 = local read "Slide"() -> (w144:i64)
        n172 = Divide(x=w139, y=10.0) -> (x/y=w142:dbl)
        n173 = Add(x=w144, y=w142) -> (x+y=w140:dbl)
        n174 = Less?(x=w140, y=w139) -> (x < y?=w141:bool)
        n175 = Select(t=w140, s=w141, f=w139) -> (s? t:f=w138:dbl)
        n176 = local write "Slide"(w138) -> ()
      }
    }
    n177 = property on="ac_time_TopData" class="Arr (strict)"("Index Values"=w119) -> ()  [unwired: 2 in, 2 out]
    n178 = property on="acquisition_time 5" class="Arr (strict)"("Index Values"=w119) -> ()  [unwired: 2 in, 2 out]
    n179 = property on="gps_lat" class="Arr (strict)"("Index Values"=w119) -> ()  [unwired: 2 in, 2 out]
    n180 = property on="gps_lon" class="Arr (strict)"("Index Values"=w119) -> ()  [unwired: 2 in, 2 out]
    "Frame actual" <- "Slide"
  }
  n181 = TDMS Open(8:w27, 11:w21) -> (0:w47:errorcluster, 3:w46:refnum<k34>)  [unwired: 5 in]
  n182 = TDMS Open(8:w28, 11:w22) -> (0:w37:errorcluster, 3:w36:refnum<k34>)  [unwired: 5 in]
  n183 = TDMS List Contents(4:w47, 7:w46) -> (0:w45:errorcluster, 2:w43:string[], 3:w44:refnum<k34>)  [unwired: 1 in, 1 out]
  n184 = TDMS List Contents(4:w37, 7:w36) -> (0:w35:errorcluster, 2:w33:string[], 3:w34:refnum<k34>)  [unwired: 1 in, 1 out]
  n185 = for {
    tunnel: w45 -> [w358]
    tunnel: w43 -> [w352] mode=indexing
    tunnel: [w355] -> w42
    shift-right: [w354] -> w41
    shift-left: w44 -> [w357]
    # "Cada caso corresponde a un instrumento/módulo de Pionero500"
    # "Lectura TDMS SubData"
    n186 = TDMS List Contents(4:w358, 6:w352, 7:w357) -> (0:w350:errorcluster, 1:w356:string[], 2:w351:string, 3:w353:refnum<k34>)
    n187 = case shown="\"Status\"" w351 {
      tunnel: w356 -> [_ w372 w416 w445 w487 w505 w542 w606 w642 w678 w714]
      tunnel: [w359 w369 w414 w440 w485 w501 w538 w602 w638 w674 w710] -> w355
      tunnel: [w360 w368 w413 w441 w484 w500 w537 w601 w637 w673 w709] -> w354
      tunnel: w351 -> [_ w371 w407 w444 w478 w504 w541 w605 w641 w677 w713]
      tunnel: w353 -> [w360 w370 w403 w443 w474 w503 w540 w604 w640 w676 w712]
      tunnel: w350 -> [w359 w373 w402 w442 w473 w502 w539 w603 w639 w675 w711]
      frame Default {
      }
      frame "Status" {
        # "Cada caso corresponde a una medida de Pionero500"
        # "Se elimina la parte decimal de acquisition time"
        n188 = Delete From Array(array=w372, index=0) -> (deleted portion=w380:string, array with subset deleted=w377:string[])  [unwired: 1 in]
        n189 = for {
          shift-right: [w392] -> w375
          shift-left: w373 -> [w396]
          shift-right: [w395] -> w376
          shift-left: w370 -> [w398]
          tunnel: w377 -> [w391] mode=indexing
          tunnel: w371 -> [w390]
          tunnel: [w388] -> w374
          i -> [w394]
          n190 = TDMS Read(0:w398, 5:w390, 7:w391, 11:w396, 12:dbl[] [] ("channel name(s) in"), 13:TRUE ("return channels in file order? (F)")) -> (4:w395:refnum<k34>, 6:w388:string, 10:w393:dbl[], 15:w392:errorcluster)  [unwired: 2 in, 2 out]
          n191 = case shown="0" w394 {
            tunnel: w393 -> [_ w399 w400 w401]
            frame Default {
            }
            frame 0 {
              "sub_ind" <- w399
            }
            frame 1 {
              "sc_ind" <- w400
            }
            frame 2 {
              "rov_states" <- w401
            }
          }
        }
        n192 = TDMS Read(0:w376, 5:w374, 7:w380, 11:w375, 12:timestamp[] [] ("Array"), 13:TRUE) -> (4:w368:refnum<k34>, 10:w362:timestamp[], 15:w369:errorcluster)  [unwired: 2 in, 3 out]
        "ac_time_SubData" <- w362
        n193 = Array Size(array=w362) -> (size(s)=w364:i32)
        n194 = for {
          tunnel: w362 -> [w385] mode=indexing
          shift-right: [w387] -> w361
          shift-left: _ -> [w386]
          n195 = To Double Precision Float(number=w385) -> (double precision float=w384:dbl)
          n196 = Round To Nearest(number=w384) -> (nearest integer value=w383:dbl)
          n197 = To Time Stamp(1:w383) -> (0:w382:timestamp)
          n198 = Build Array (concatenate)(w386, w382) -> (w387:timestamp[])
        }
        "round_ac_time_SubData" <- w361
        n199 = Decrement(x=w364) -> (x-1=w363:i32)
        n200 = Index Array(array=w362, index=0) -> (element=→"inicio_SubData":timestamp)
        n201 = Index Array(array=w362, index=w363) -> (element=→"fin_SubData":timestamp)
      }
      frame "AHRS" {
        # "Cada caso corresponde a una medida de Pionero500"
        n202 = Delete From Array(array=w416, index=0) -> (deleted portion=w412:string, array with subset deleted=w408:string[])  [unwired: 1 in]
        n203 = for {
          shift-right: [w421] -> w405
          shift-left: w402 -> [w425]
          shift-right: [w424] -> w406
          shift-left: w403 -> [w427]
          tunnel: w408 -> [w420] mode=indexing
          tunnel: w407 -> [w419]
          tunnel: [w417] -> w404
          i -> [w423]
          n204 = TDMS Read(0:w427, 5:w419, 7:w420, 11:w425, 12:dbl[] [] ("channel name(s) in"), 13:TRUE ("return channels in file order? (F)")) -> (4:w424:refnum<k34>, 6:w417:string, 10:w422:dbl[], 15:w421:errorcluster)  [unwired: 2 in, 2 out]
          n205 = case shown="1" w423 {
            tunnel: w422 -> [_ w428 w429 w430 w431 w432 w433 w434 w435 w436 w437 w438 w439]
            frame Default {
            }
            frame 0 {
              "pitch" <- w428
            }
            frame 1 {
              "roll" <- w429
            }
            frame 2 {
              "heading" <- w430
            }
            frame 3 {
              "accel_x" <- w431
            }
            frame 4 {
              "accel_y" <- w432
            }
            frame 5 {
              "accel_z" <- w433
            }
            frame 6 {
              "gyr_x" <- w434
            }
            frame 7 {
              "gyr_y" <- w435
            }
            frame 8 {
              "gyr_z" <- w436
            }
            frame 9 {
              "mag_x" <- w437
            }
            frame 10 {
              "mag_y" <- w438
            }
            frame 11 {
              "mag_z" <- w439
            }
          }
        }
        n206 = TDMS Read(0:w406, 5:w404, 7:w412, 11:w405, 12:timestamp[] [] ("Array"), 13:TRUE) -> (4:w413:refnum<k34>, 10:→"acquisition_time 2":timestamp[], 15:w414:errorcluster)  [unwired: 2 in, 3 out]
      }
      frame "CTD" {
        # "Cada caso corresponde a una medida de Pionero500"
        n207 = Delete From Array(array=w445, index=0) -> (deleted portion=w449:string, array with subset deleted=w451:string[])  [unwired: 1 in]
        n208 = for {
          shift-right: [w459] -> w453
          shift-left: w442 -> [w463]
          shift-right: [w462] -> w452
          shift-left: w443 -> [w465]
          tunnel: w451 -> [w458] mode=indexing
          tunnel: w444 -> [w457]
          tunnel: [w455] -> w454
          i -> [w461]
          n209 = TDMS Read(0:w465, 5:w457, 7:w458, 11:w463, 12:dbl[] [] ("channel name(s) in"), 13:TRUE ("return channels in file order? (F)")) -> (4:w462:refnum<k34>, 6:w455:string, 10:w460:dbl[], 15:w459:errorcluster)  [unwired: 2 in, 2 out]
          n210 = case shown="6" w461 {
            tunnel: w460 -> [_ w466 w467 w468 w469 w470 w471 w472]
            frame Default {
            }
            frame 0 {
              "pressure 4" <- w466
            }
            frame 1 {
              "temperature 4" <- w467
            }
            frame 2 {
              "conductivity" <- w468
            }
            frame 3 {
              "density" <- w469
            }
            frame 4 {
              "salinity" <- w470
            }
            frame 5 {
              "speed_of_sound" <- w471
            }
            frame 6 {
              "depth" <- w472
            }
          }
        }
        n211 = TDMS Read(0:w452, 5:w454, 7:w449, 11:w453, 12:timestamp[] [] ("Array"), 13:TRUE) -> (4:w441:refnum<k34>, 10:→"acquisition_time 4":timestamp[], 15:w440:errorcluster)  [unwired: 2 in, 3 out]
      }
      frame "ALTIMETER" {
        # "Cada caso corresponde a una medida de Pionero500"
        n212 = Delete From Array(array=w487, index=0) -> (deleted portion=w483:string, array with subset deleted=w479:string[])  [unwired: 1 in]
        n213 = for {
          shift-right: [w492] -> w476
          shift-left: w473 -> [w496]
          shift-right: [w495] -> w477
          shift-left: w474 -> [w498]
          tunnel: w479 -> [w491] mode=indexing
          tunnel: w478 -> [w490]
          tunnel: [w488] -> w475
          i -> [w494]
          n214 = TDMS Read(0:w498, 5:w490, 7:w491, 11:w496, 12:dbl[] [] ("channel name(s) in"), 13:TRUE ("return channels in file order? (F)")) -> (4:w495:refnum<k34>, 6:w488:string, 10:w493:dbl[], 15:w492:errorcluster)  [unwired: 2 in, 2 out]
          n215 = case shown="0" w494 {
            tunnel: w493 -> [_ w499]
            frame Default {
            }
            frame 0 {
              "altitude" <- w499
            }
          }
        }
        n216 = TDMS Read(0:w477, 5:w475, 7:w483, 11:w476, 12:timestamp[] [] ("Array"), 13:TRUE) -> (4:w484:refnum<k34>, 10:→"acquisition_time 3":timestamp[], 15:w485:errorcluster)  [unwired: 2 in, 3 out]
      }
      frame "SMP" {
        # "Cada caso corresponde a una medida de Pionero500"
        n217 = Delete From Array(array=w505, index=0) -> (deleted portion=w513:string, array with subset deleted=w509:string[])  [unwired: 1 in]
        n218 = for {
          shift-right: [w519] -> w507
          shift-left: w502 -> [w523]
          shift-right: [w522] -> w508
          shift-left: w503 -> [w525]
          tunnel: w509 -> [w518] mode=indexing
          tunnel: w504 -> [w517]
          tunnel: [w515] -> w506
          i -> [w521]
          n219 = TDMS Read(0:w525, 5:w517, 7:w518, 11:w523, 12:dbl[] [] ("channel name(s) in"), 13:TRUE ("return channels in file order? (F)")) -> (4:w522:refnum<k34>, 6:w515:string, 10:w520:dbl[], 15:w519:errorcluster)  [unwired: 2 in, 2 out]
          n220 = case shown="0" w521 {
            tunnel: w520 -> [_ w526 w527 w528 w529 w530 w531 w532 w533 w534 w535 w536]
            frame Default {
            }
            frame 0 {
              "liquid_smp1" <- w526
            }
            frame 1 {
              "liquid_smp2" <- w527
            }
            frame 2 {
              "liquid_smp3" <- w528
            }
            frame 3 {
              "liquid_smp4" <- w529
            }
            frame 4 {
              "solid_smp1" <- w530
            }
            frame 5 {
              "solid_smp2" <- w531
            }
            frame 6 {
              "supply_12V" <- w532
            }
            frame 7 {
              "motor_signal1" <- w533
            }
            frame 8 {
              "motor_signal2" <- w534
            }
            frame 9 {
              "cur_liq_1" <- w535
            }
            frame 10 {
              "cur_liq_2" <- w536
            }
          }
        }
        n221 = TDMS Read(0:w508, 5:w506, 7:w513, 11:w507, 12:timestamp[] [] ("Array"), 13:TRUE) -> (4:w500:refnum<k34>, 10:→"acquisition_time 6":timestamp[], 15:w501:errorcluster)  [unwired: 2 in, 3 out]
      }
      frame "PWR" {
        # "Cada caso corresponde a una medida de Pionero500"
        n222 = Delete From Array(array=w542, index=0) -> (deleted portion=w550:string, array with subset deleted=w546:string[])  [unwired: 1 in]
        n223 = for {
          shift-right: [w556] -> w544
          shift-left: w539 -> [w560]
          shift-right: [w559] -> w545
          shift-left: w540 -> [w562]
          tunnel: w546 -> [w555] mode=indexing
          tunnel: w541 -> [w554]
          tunnel: [w552] -> w543
          i -> [w558]
          n224 = TDMS Read(0:w562, 5:w554, 7:w555, 11:w560, 12:dbl[] [] ("channel name(s) in"), 13:TRUE ("return channels in file order? (F)")) -> (4:w559:refnum<k34>, 6:w552:string, 10:w557:dbl[], 15:w556:errorcluster)  [unwired: 2 in, 2 out]
          n225 = case shown="12" w558 {
            tunnel: w557 -> [_ w563 w564 w565 w566 w567 w568 w569 w570 w571 w572 w573 w574 w575 w576 w577 w578 w579 w580 w581 w582 w583 w584 w585 w586 w587 w588 w589 w590 w591 w592 w593 w594 w595 w596 w597 w598 w599 w600]
            frame Default {
            }
            frame 0 {
              "ac_status" <- w563
            }
            frame 1 {
              "voltaje_hvdc" <- w564
            }
            frame 2 {
              "current_hvdc" <- w565
            }
            frame 3 {
              "light1" <- w566
            }
            frame 4 {
              "light2" <- w567
            }
            frame 5 {
              "ligth_sphere" <- w568
            }
            frame 6 {
              "voltage_l1_l2" <- w569
            }
            frame 7 {
              "voltage_l2_l3" <- w570
            }
            frame 8 {
              "voltage_l1_l3" <- w571
            }
            frame 9 {
              "current_l1" <- w572
            }
            frame 10 {
              "current_l2" <- w573
            }
            frame 11 {
              "current_l3" <- w574
            }
            frame 12 {
              "current_lights" <- w575
            }
            frame 13 {
              "temp_ac_filter" <- w576
            }
            frame 14 {
              "MA_1_status" <- w577
            }
            frame 15 {
              "MA_1_ctr_signal" <- w578
            }
            frame 16 {
              "MA_1_current" <- w579
            }
            frame 17 {
              "MA_1_speed" <- w580
            }
            frame 18 {
              "MA_2_status" <- w581
            }
            frame 19 {
              "MA_2_ctr_signal" <- w582
            }
            frame 20 {
              "MA_2_current" <- w583
            }
            frame 21 {
              "MA_2_speed" <- w584
            }
            frame 22 {
              "MA_3_status" <- w585
            }
            frame 23 {
              "MA_3_ctr_signal" <- w586
            }
            frame 24 {
              "MA_3_current" <- w587
            }
            frame 25 {
              "MA_3_speed" <- w588
            }
            frame 26 {
              "MA_4_status" <- w589
            }
            frame 27 {
              "MA_4_ctr_signal" <- w590
            }
            frame 28 {
              "MA_4_current" <- w591
            }
            frame 29 {
              "MA_4_speed" <- w592
            }
            frame 30 {
              "MA_5_status" <- w593
            }
            frame 31 {
              "MA_5_ctr_signal" <- w594
            }
            frame 32 {
              "MA_5_current" <- w595
            }
            frame 33 {
              "MA_5_speed" <- w596
            }
            frame 34 {
              "MA_6_status" <- w597
            }
            frame 35 {
              "MA_6_ctr_signal" <- w598
            }
            frame 36 {
              "MA_6_current" <- w599
            }
            frame 37 {
              "MA_6_speed" <- w600
            }
          }
        }
        n226 = TDMS Read(0:w545, 5:w543, 7:w550, 11:w544, 12:timestamp[] [] ("Array"), 13:TRUE) -> (4:w537:refnum<k34>, 10:→"acquisition_time 7":timestamp[], 15:w538:errorcluster)  [unwired: 2 in, 3 out]
      }
      frame "SC_PWR" {
        # "Cada caso corresponde a una medida de Pionero500"
        n227 = Delete From Array(array=w606, index=0) -> (deleted portion=w614:string, array with subset deleted=w610:string[])  [unwired: 1 in]
        n228 = for {
          shift-right: [w620] -> w608
          shift-left: w603 -> [w624]
          shift-right: [w623] -> w609
          shift-left: w604 -> [w626]
          tunnel: w610 -> [w619] mode=indexing
          tunnel: w605 -> [w618]
          tunnel: [w616] -> w607
          i -> [w622]
          n229 = TDMS Read(0:w626, 5:w618, 7:w619, 11:w624, 12:dbl[] [] ("channel name(s) in"), 13:TRUE ("return channels in file order? (F)")) -> (4:w623:refnum<k34>, 6:w616:string, 10:w621:dbl[], 15:w620:errorcluster)  [unwired: 2 in, 2 out]
          n230 = case shown="0" w622 {
            tunnel: w621 -> [_ w627 w628 w629 w630 w631 w632 w633 w634 w635 w636]
            frame Default {
            }
            frame 0 {
              "mode" <- w627
            }
            frame 1 {
              "start" <- w628
            }
            frame 2 {
              "lps" <- w629
            }
            frame 3 {
              "controller" <- w630
            }
            frame 4 {
              "voltage" <- w631
            }
            frame 5 {
              "current" <- w632
            }
            frame 6 {
              "temperature" <- w633
            }
            frame 7 {
              "humidity" <- w634
            }
            frame 8 {
              "leak" <- w635
            }
            frame 9 {
              "pressure" <- w636
            }
          }
        }
        n231 = TDMS Read(0:w609, 5:w607, 7:w614, 11:w608, 12:timestamp[] [] ("Array"), 13:TRUE) -> (4:w601:refnum<k34>, 10:→"acquisition_time 8":timestamp[], 15:w602:errorcluster)  [unwired: 2 in, 3 out]
      }
      frame "SC_CPU" {
        # "Cada caso corresponde a una medida de Pionero500"
        n232 = Delete From Array(array=w642, index=0) -> (deleted portion=w650:string, array with subset deleted=w646:string[])  [unwired: 1 in]
        n233 = for {
          shift-right: [w656] -> w644
          shift-left: w639 -> [w660]
          shift-right: [w659] -> w645
          shift-left: w640 -> [w662]
          tunnel: w646 -> [w655] mode=indexing
          tunnel: w641 -> [w654]
          tunnel: [w652] -> w643
          i -> [w658]
          n234 = TDMS Read(0:w662, 5:w654, 7:w655, 11:w660, 12:dbl[] [] ("channel name(s) in"), 13:TRUE ("return channels in file order? (F)")) -> (4:w659:refnum<k34>, 6:w652:string, 10:w657:dbl[], 15:w656:errorcluster)  [unwired: 2 in, 2 out]
          n235 = case shown="0" w658 {
            tunnel: w657 -> [_ w663 w664 w665 w666 w667 w668 w669 w670 w671 w672]
            frame Default {
            }
            frame 0 {
              "mode 2" <- w663
            }
            frame 1 {
              "start 2" <- w664
            }
            frame 2 {
              "lps 2" <- w665
            }
            frame 3 {
              "controller 2" <- w666
            }
            frame 4 {
              "voltage 2" <- w667
            }
            frame 5 {
              "current 2" <- w668
            }
            frame 6 {
              "temperature 2" <- w669
            }
            frame 7 {
              "humidity 2" <- w670
            }
            frame 8 {
              "leak 2" <- w671
            }
            frame 9 {
              "pressure 2" <- w672
            }
          }
        }
        n236 = TDMS Read(0:w645, 5:w643, 7:w650, 11:w644, 12:timestamp[] [] ("Array"), 13:TRUE) -> (4:w637:refnum<k34>, 10:→"acquisition_time 9":timestamp[], 15:w638:errorcluster)  [unwired: 2 in, 3 out]
      }
      frame "SC_SMP" {
        # "Cada caso corresponde a una medida de Pionero500"
        n237 = Delete From Array(array=w678, index=0) -> (deleted portion=w686:string, array with subset deleted=w682:string[])  [unwired: 1 in]
        n238 = for {
          shift-right: [w692] -> w680
          shift-left: w675 -> [w696]
          shift-right: [w695] -> w681
          shift-left: w676 -> [w698]
          tunnel: w682 -> [w691] mode=indexing
          tunnel: w677 -> [w690]
          tunnel: [w688] -> w679
          i -> [w694]
          n239 = TDMS Read(0:w698, 5:w690, 7:w691, 11:w696, 12:dbl[] [] ("channel name(s) in"), 13:TRUE ("return channels in file order? (F)")) -> (4:w695:refnum<k34>, 6:w688:string, 10:w693:dbl[], 15:w692:errorcluster)  [unwired: 2 in, 2 out]
          n240 = case shown="0" w694 {
            tunnel: w693 -> [_ w699 w700 w701 w702 w703 w704 w705 w706 w707 w708]
            frame Default {
            }
            frame 0 {
              "mode 3" <- w699
            }
            frame 1 {
              "start 3" <- w700
            }
            frame 2 {
              "lps 3" <- w701
            }
            frame 3 {
              "controller 3" <- w702
            }
            frame 4 {
              "voltage 3" <- w703
            }
            frame 5 {
              "current 3" <- w704
            }
            frame 6 {
              "temperature 3" <- w705
            }
            frame 7 {
              "humidity 3" <- w706
            }
            frame 8 {
              "leak 3" <- w707
            }
            frame 9 {
              "pressure 3" <- w708
            }
          }
        }
        n241 = TDMS Read(0:w681, 5:w679, 7:w686, 11:w680, 12:timestamp[] [] ("Array"), 13:TRUE) -> (4:w673:refnum<k34>, 10:→"acquisition_time 10":timestamp[], 15:w674:errorcluster)  [unwired: 2 in, 3 out]
      }
      frame "Control" {
        # "Cada caso corresponde a una medida de Pionero500"
        n242 = Delete From Array(array=w714, index=0) -> (deleted portion=w722:string, array with subset deleted=w718:string[])  [unwired: 1 in]
        n243 = for {
          shift-right: [w728] -> w716
          shift-left: w711 -> [w732]
          shift-right: [w731] -> w717
          shift-left: w712 -> [w734]
          tunnel: w718 -> [w727] mode=indexing
          tunnel: w713 -> [w726]
          tunnel: [w724] -> w715
          i -> [w730]
          n244 = TDMS Read(0:w734, 5:w726, 7:w727, 11:w732, 12:dbl[] [] ("channel name(s) in"), 13:TRUE ("return channels in file order? (F)")) -> (4:w731:refnum<k34>, 6:w724:string, 10:w729:dbl[], 15:w728:errorcluster)  [unwired: 2 in, 2 out]
          n245 = case shown="0" w730 {
            tunnel: w729 -> [_ w735 w736 w737 w738 w739 w740 w741 w742 w743]
            frame Default {
            }
            frame 0 {
              "ctrl_state" <- w735
            }
            frame 1 {
              "rov_output_x" <- w736
            }
            frame 2 {
              "rov_output_y" <- w737
            }
            frame 3 {
              "rov_output_z" <- w738
            }
            frame 4 {
              "rov_output_yaw" <- w739
            }
            frame 5 {
              "dac_outputs" <- w740
            }
            frame 6 {
              "in_range" <- w741
            }
            frame 7 {
              "motor_ctrl_array_setpoint" <- w742
            }
            frame 8 {
              "motor_ctrl_array_sensor" <- w743
            }
          }
        }
        n246 = TDMS Read(0:w717, 5:w715, 7:w722, 11:w716, 12:timestamp[] [] ("Array"), 13:TRUE) -> (4:w709:refnum<k34>, 10:→"acquisition_time 11":timestamp[], 15:w710:errorcluster)  [unwired: 2 in, 3 out]
      }
    }
  }
  n247 = for {
    tunnel: w35 -> [w752]
    tunnel: w33 -> [w746] mode=indexing
    tunnel: [w749] -> w32
    shift-right: [w748] -> w31
    shift-left: w34 -> [w751]
    # "Cada caso corresponde a un instrumento/módulo de Pionero500"
    # "Lectura TDMS TopData"
    n248 = TDMS List Contents(4:w752, 6:w746, 7:w751) -> (0:w744:errorcluster, 1:w750:string[], 2:w745:string, 3:w747:refnum<k34>)
    n249 = case shown="\"Status\"" w745 {
      tunnel: w750 -> [_ w766 w810 w836 w915 w971]
      tunnel: [w753 w763 w808 w831 w913 w969] -> w749
      tunnel: [w754 w762 w807 w832 w912 w968] -> w748
      tunnel: w745 -> [_ w765 w801 w835 w906 w962]
      tunnel: w747 -> [w754 w764 w797 w834 w902 w958]
      tunnel: w744 -> [w753 w767 w796 w833 w901 w957]
      frame Default {
      }
      frame "Status" {
        # "Cada caso corresponde a una medida de Pionero500"
        # "Se elimina la parte decimal de acquisition time"
        n250 = Delete From Array(array=w766, index=0) -> (deleted portion=w774:string, array with subset deleted=w771:string[])  [unwired: 1 in]
        n251 = for {
          shift-right: [w786] -> w769
          shift-left: w767 -> [w790]
          shift-right: [w789] -> w770
          shift-left: w764 -> [w792]
          tunnel: w771 -> [w785] mode=indexing
          tunnel: w765 -> [w784]
          tunnel: [w782] -> w768
          i -> [w788]
          n252 = TDMS Read(0:w792, 5:w784, 7:w785, 11:w790, 12:dbl[] [] ("channel name(s) in"), 13:TRUE ("return channels in file order? (F)")) -> (4:w789:refnum<k34>, 6:w782:string, 10:w787:dbl[], 15:w786:errorcluster)  [unwired: 2 in, 2 out]
          n253 = case shown="0" w788 {
            tunnel: w787 -> [_ w793 w794 w795]
            frame Default {
            }
            frame 0 {
              "rov_states 2" <- w793
            }
            frame 1 {
              "ind." <- w794
            }
            frame 2 {
              "modo_ctrl 2" <- w795
            }
          }
        }
        n254 = TDMS Read(0:w770, 5:w768, 7:w774, 11:w769, 12:timestamp[] [] ("Array"), 13:TRUE) -> (4:w762:refnum<k34>, 10:w755:timestamp[], 15:w763:errorcluster)  [unwired: 2 in, 3 out]
        "ac_time_TopData" <- w755
        n255 = Array Size(array=w755) -> (size(s)=w758:i32)
        n256 = for {
          tunnel: w755 -> [w779] mode=indexing
          shift-right: [w781] -> w756
          shift-left: _ -> [w780]
          n257 = To Double Precision Float(number=w779) -> (double precision float=w778:dbl)
          n258 = Round To Nearest(number=w778) -> (nearest integer value=w777:dbl)
          n259 = To Time Stamp(1:w777) -> (0:w776:timestamp)
          n260 = Build Array (concatenate)(w780, w776) -> (w781:timestamp[])
        }
        "round_ac_time_TopData" <- w756
        n261 = Decrement(x=w758) -> (x-1=w757:i32)
        n262 = Index Array(array=w755, index=0) -> (element=→"inicio_TopData":timestamp)
        n263 = Index Array(array=w755, index=w757) -> (element=→"fin_TopData":timestamp)
      }
      frame "DAQ" {
        # "Cada caso corresponde a una medida de Pionero500"
        n264 = Delete From Array(array=w810, index=0) -> (deleted portion=w806:string, array with subset deleted=w802:string[])  [unwired: 1 in]
        n265 = for {
          shift-right: [w815] -> w799
          shift-left: w796 -> [w819]
          shift-right: [w818] -> w800
          shift-left: w797 -> [w821]
          tunnel: w802 -> [w814] mode=indexing
          tunnel: w801 -> [w813]
          tunnel: [w811] -> w798
          i -> [w817]
          n266 = TDMS Read(0:w821, 5:w813, 7:w814, 11:w819, 12:dbl[] [] ("channel name(s) in"), 13:TRUE ("return channels in file order? (F)")) -> (4:w818:refnum<k34>, 6:w811:string, 10:w816:dbl[], 15:w815:errorcluster)  [unwired: 2 in, 2 out]
          n267 = case shown="0" w817 {
            tunnel: w816 -> [_ w822 w823 w824 w825 w826 w827 w828 w829 w830]
            frame Default {
            }
            frame 0 {
              "gps_lat" <- w822
            }
            frame 1 {
              "gps_lon" <- w823
            }
            frame 2 {
              "gps_alt" <- w824
            }
            frame 3 {
              "usbl_x" <- w825
            }
            frame 4 {
              "usbl_y" <- w826
            }
            frame 5 {
              "usbl_z" <- w827
            }
            frame 6 {
              "vess_ahrs_pitch" <- w828
            }
            frame 7 {
              "vess_ahrs_roll" <- w829
            }
            frame 8 {
              "vess_ahrs_yaw" <- w830
            }
          }
        }
        n268 = TDMS Read(0:w800, 5:w798, 7:w806, 11:w799, 12:timestamp[] [] ("Array"), 13:TRUE) -> (4:w807:refnum<k34>, 10:→"acquisition_time 5":timestamp[], 15:w808:errorcluster)  [unwired: 2 in, 3 out]
      }
      frame "User_Data" {
        # "Cada caso corresponde a una medida de Pionero500"
        n269 = Delete From Array(array=w836, index=0) -> (deleted portion=w840:string, array with subset deleted=w842:string[])  [unwired: 1 in]
        n270 = for {
          shift-right: [w850] -> w844
          shift-left: w833 -> [w854]
          shift-right: [w853] -> w843
          shift-left: w834 -> [w856]
          tunnel: w842 -> [w849] mode=indexing
          tunnel: w835 -> [w848]
          tunnel: [w846] -> w845
          i -> [w852]
          n271 = TDMS Read(0:w856, 5:w848, 7:w849, 11:w854, 12:dbl[] [] ("channel name(s) in"), 13:TRUE ("return channels in file order? (F)")) -> (4:w853:refnum<k34>, 6:w846:string, 10:w851:dbl[], 15:w850:errorcluster)  [unwired: 2 in, 2 out]
          n272 = case shown="1" w852 {
            tunnel: w851 -> [_ w857 w858 w859 w860 w861 w862 w863 w864 w865 w866 w867 w868 w869 w870 w871 w872 w873 w874 w875 w876 w877 w878 w879 w880 w881 w882 w883 w884 w885 w886 w887 w888 w889 w890 w891 w892 w893 w894 w895 w896 w897 w898 w899 w900]
            frame Default {
            }
            frame 0 {
              "ci_habilitada" <- w857
            }
            frame 1 {
              "CI_Data_joy_1x" <- w858
            }
            frame 2 {
              "CI_Data_jot_1y" <- w859
            }
            frame 3 {
              "CI_Data_jot_1z" <- w860
            }
            frame 4 {
              "CI_Data_joy_1thumb" <- w861
            }
            frame 5 {
              "CI_Data_joy_1botIzq" <- w862
            }
            frame 6 {
              "CI_Data_joy_1botder" <- w863
            }
            frame 7 {
              "CI_Data_joy_1gatillo" <- w864
            }
            frame 8 {
              "CI_Data_modo_1bot" <- w865
            }
            frame 9 {
              "CI_Data_modo_2bot" <- w866
            }
            frame 10 {
              "CI_Data_modo_3bot" <- w867
            }
            frame 11 {
              "CI_Data_modo_4bot" <- w868
            }
            frame 12 {
              "CI_Data_pot" <- w869
            }
            frame 13 {
              "CI_Data_enc" <- w870
            }
            frame 14 {
              "CI_Data_joy_2x" <- w871
            }
            frame 15 {
              "CI_Data_joy_2y" <- w872
            }
            frame 16 {
              "CI_Data_joy_2z" <- w873
            }
            frame 17 {
              "CI_Data_joy_2bot" <- w874
            }
            frame 18 {
              "CI_Data_botella_1bot" <- w875
            }
            frame 19 {
              "CI_Data_botella_2bot" <- w876
            }
            frame 20 {
              "CI_Data_botella_3bot" <- w877
            }
            frame 21 {
              "CI_Data_botella_4bot" <- w878
            }
            frame 22 {
              "CI_Data_corer_1bot" <- w879
            }
            frame 23 {
              "CI_Data_corer_2bot" <- w880
            }
            frame 24 {
              "CI_Data_a_in" <- w881
            }
            frame 25 {
              "CI_Data_dio1" <- w882
            }
            frame 26 {
              "CI_Data_dio2" <- w883
            }
            frame 27 {
              "CI_Data_dio3" <- w884
            }
            frame 28 {
              "CI_Data_ci_acc_x" <- w885
            }
            frame 29 {
              "CI_Data_ci_acc_y" <- w886
            }
            frame 30 {
              "CI_Data_ci_acc_z" <- w887
            }
            frame 31 {
              "Surface_Data_modo_1ind" <- w888
            }
            frame 32 {
              "Surface_Data_modo_2ind" <- w889
            }
            frame 33 {
              "Surface_Data_modo_3ind" <- w890
            }
            frame 34 {
              "Surface_Data_modo_4ind" <- w891
            }
            frame 35 {
              "Surface_Data_botella_1ind" <- w892
            }
            frame 36 {
              "Surface_Data_botella_2ind" <- w893
            }
            frame 37 {
              "Surface_Data_botella_3ind" <- w894
            }
            frame 38 {
              "Surface_Data_botella_4ind" <- w895
            }
            frame 39 {
              "Surface_Data_corer_1ind" <- w896
            }
            frame 40 {
              "Surface_Data_corer_2ind" <- w897
            }
            frame 41 {
              "Surface_Data_lars_vel" <- w898
            }
            frame 42 {
              "Surface_Data_lars_fwd" <- w899
            }
            frame 43 {
              "Surface_Data_lars_rev" <- w900
            }
          }
        }
        n273 = TDMS Read(0:w843, 5:w845, 7:w840, 11:w844, 12:timestamp[] [] ("Array"), 13:TRUE) -> (4:w832:refnum<k34>, 10:→"acquisition_time 12":timestamp[], 15:w831:errorcluster)  [unwired: 2 in, 3 out]
      }
      frame "Virtual_CI" {
        # "Cada caso corresponde a una medida de Pionero500"
        n274 = Delete From Array(array=w915, index=0) -> (deleted portion=w911:string, array with subset deleted=w907:string[])  [unwired: 1 in]
        n275 = for {
          shift-right: [w922] -> w904
          shift-left: w901 -> [w924]
          shift-right: [w923] -> w905
          shift-left: w902 -> [w926]
          tunnel: w907 -> [w921] mode=indexing
          tunnel: w906 -> [w920]
          tunnel: [w918] -> w903
          i -> [w917]
          n276 = TDMS Read(0:w926, 5:w920, 7:w921, 11:w924, 12:dbl[] [] ("channel name(s) in"), 13:TRUE ("return channels in file order? (F)")) -> (4:w923:refnum<k34>, 6:w918:string, 10:w916:dbl[], 15:w922:errorcluster)  [unwired: 2 in, 2 out]
          n277 = case shown="0" w917 {
            tunnel: w916 -> [_ w927 w928 w929 w930 w931 w932 w933 w934 w935 w936 w937 w938 w939 w940 w941 w942 w943 w944 w945 w946 w947 w948 w949 w950 w951 w952 w953 w954 w955 w956]
            frame Default {
            }
            frame 0 {
              "bus_260v" <- w927
            }
            frame 1 {
              "m_1" <- w928
            }
            frame 2 {
              "m_2" <- w929
            }
            frame 3 {
              "m_3" <- w930
            }
            frame 4 {
              "m_4" <- w931
            }
            frame 5 {
              "m_5" <- w932
            }
            frame 6 {
              "m_6" <- w933
            }
            frame 7 {
              "luz_1" <- w934
            }
            frame 8 {
              "luz_2" <- w935
            }
            frame 9 {
              "luz_3" <- w936
            }
            frame 10 {
              "pot_gen" <- w937
            }
            frame 11 {
              "pot_m1" <- w938
            }
            frame 12 {
              "pot_m2" <- w939
            }
            frame 13 {
              "pot_m3" <- w940
            }
            frame 14 {
              "pot_m4" <- w941
            }
            frame 15 {
              "pot_m5" <- w942
            }
            frame 16 {
              "pot_m6" <- w943
            }
            frame 17 {
              "pot_l1" <- w944
            }
            frame 18 {
              "pot_l2" <- w945
            }
            frame 19 {
              "pot_l3" <- w946
            }
            frame 20 {
              "virtual_ci" <- w947
            }
            frame 21 {
              "fuente_muestras" <- w948
            }
            frame 22 {
              "corer_1" <- w949
            }
            frame 23 {
              "corer_2" <- w950
            }
            frame 24 {
              "bot_1" <- w951
            }
            frame 25 {
              "bot_2" <- w952
            }
            frame 26 {
              "bot_3" <- w953
            }
            frame 27 {
              "bot_4" <- w954
            }
            frame 28 {
              "pot_c1" <- w955
            }
            frame 29 {
              "pot_c2" <- w956
            }
          }
        }
        n278 = TDMS Read(0:w905, 5:w903, 7:w911, 11:w904, 12:timestamp[] [] ("Array"), 13:TRUE) -> (4:w912:refnum<k34>, 10:→"acquisition_time 13":timestamp[], 15:w913:errorcluster)  [unwired: 2 in, 3 out]
      }
      frame "Control" {
        # "Cada caso corresponde a una medida de Pionero500"
        n279 = Delete From Array(array=w971, index=0) -> (deleted portion=w967:string, array with subset deleted=w963:string[])  [unwired: 1 in]
        n280 = for {
          shift-right: [w978] -> w960
          shift-left: w957 -> [w980]
          shift-right: [w979] -> w961
          shift-left: w958 -> [w982]
          tunnel: w963 -> [w977] mode=indexing
          tunnel: w962 -> [w976]
          tunnel: [w974] -> w959
          i -> [w973]
          n281 = TDMS Read(0:w982, 5:w976, 7:w977, 11:w980, 12:dbl[] [] ("channel name(s) in"), 13:TRUE ("return channels in file order? (F)")) -> (4:w979:refnum<k34>, 6:w974:string, 10:w972:dbl[], 15:w978:errorcluster)  [unwired: 2 in, 2 out]
          n282 = case shown="0" w973 {
            tunnel: w972 -> [_ w983 w984 w985 w986 w987 w988 w989 w990 w991 w992 w993 w994 w995 w996 w997 w998 w999 w1000 w1001 w1002 w1003 w1004 w1005 w1006 w1007 w1008 w1009 w1010 w1011 w1012 w1013 w1014 w1015 w1016 w1017 w1018]
            frame Default {
            }
            frame 0 {
              "m1_hi" <- w983
            }
            frame 1 {
              "m1_lo" <- w984
            }
            frame 2 {
              "m1_en" <- w985
            }
            frame 3 {
              "m2_hi" <- w986
            }
            frame 4 {
              "m2_lo" <- w987
            }
            frame 5 {
              "m2_en" <- w988
            }
            frame 6 {
              "m3_hi" <- w989
            }
            frame 7 {
              "m3_lo" <- w990
            }
            frame 8 {
              "m3_en" <- w991
            }
            frame 9 {
              "m4_hi" <- w992
            }
            frame 10 {
              "m4_lo" <- w993
            }
            frame 11 {
              "m4_en" <- w994
            }
            frame 12 {
              "m5_hi" <- w995
            }
            frame 13 {
              "m5_lo" <- w996
            }
            frame 14 {
              "m5_en" <- w997
            }
            frame 15 {
              "m6_hi" <- w998
            }
            frame 16 {
              "m6_lo" <- w999
            }
            frame 17 {
              "m6_en" <- w1000
            }
            frame 18 {
              "motor_PID_Kp" <- w1001
            }
            frame 19 {
              "motor_PID_Ti" <- w1002
            }
            frame 20 {
              "motor_PID_Td" <- w1003
            }
            frame 21 {
              "m_PID_en" <- w1004
            }
            frame 22 {
              "depth_PID_Kp" <- w1005
            }
            frame 23 {
              "depth_PID_Ti" <- w1006
            }
            frame 24 {
              "depth_PID_Td" <- w1007
            }
            frame 25 {
              "depth_sp" <- w1008
            }
            frame 26 {
              "heading_PID_Kp" <- w1009
            }
            frame 27 {
              "heading_PID_Ti" <- w1010
            }
            frame 28 {
              "heading_PID_Td" <- w1011
            }
            frame 29 {
              "heading_sp" <- w1012
            }
            frame 30 {
              "altitude_PID_Kp" <- w1013
            }
            frame 31 {
              "altitude_PID_Ti" <- w1014
            }
            frame 32 {
              "altitude_PID_Td" <- w1015
            }
            frame 33 {
              "altitude_sp" <- w1016
            }
            frame 34 {
              "PID_reset" <- w1017
            }
            frame 35 {
              "modo_ctrl" <- w1018
            }
          }
        }
        n283 = TDMS Read(0:w961, 5:w959, 7:w967, 11:w960, 12:timestamp[] [] ("Array"), 13:TRUE) -> (4:w968:refnum<k34>, 10:→"acquisition_time 14":timestamp[], 15:w969:errorcluster)  [unwired: 2 in, 3 out]
      }
    }
  }
  n284 = TDMS Close(8:w32, 11:w31) -> (0:w24:errorcluster)  [unwired: 1 out]
  n285 = TDMS Close(8:w42, 11:w41) -> (0:w23:errorcluster)  [unwired: 1 out]
  n286 = call "IMAQ AVI Close"("Avi Refnum"=w63) -> ("error out"=w50:errorcluster)  [unwired: 10 in]
  n287 = call "IMAQ Dispose"("Image"=w60, "error in (no error)"=w4) -> ("error out"=w51:errorcluster)  [unwired: 4 in]
  n288 = Merge Errors(w24, w23, w50, w51) -> (w49:errorcluster)
  n289 = flat-sequence {
    tunnel: w49 -> [w1019]
    frame #0 {
      n290 = call <vilib>:"Simple Error Handler.vi"("error in (no error)"=w1019) -> ()  [unwired: 4 in, 5 out]
    }
  }
  "is_gps_lat" <- w2
  "is_gps_lon" <- w2
  "is_pitch" <- w2
  "is_roll" <- w2
  "is_heading" <- w2
  "is_altitude" <- w2
  "is_depth" <- w2
